vi "Elbow Call.vi"(3 "Button Values":bool[](array[boolean])) -> ()   [LabVIEW 2018]
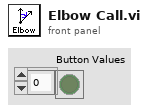
[diagram p1: front panel]
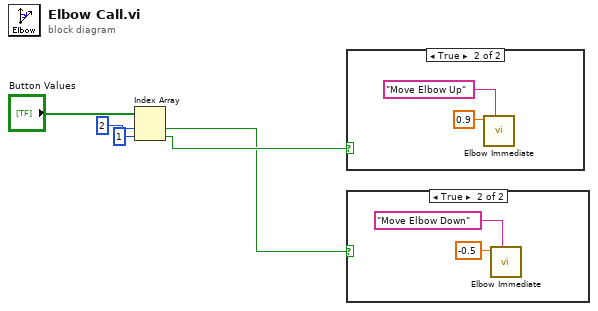
[diagram p0: block diagram]
diagram:
  n1 = Index Array(array="Button Values", index #1=2 ("index"), index #2=1 ("index")) -> (element #1=w1:bool, element #2=w2:bool)
  n2 = case shown="True" w2 {
    frame False {
    }
    frame True {
      n3 = call "Elbow Immediate.vi"("Description"="Move Elbow Up", "Setpoint"=0.9) -> ()  [unwired: 9 in, 1 out]
    }
  }
  n4 = case shown="True" w1 {
    frame False {
    }
    frame True {
      n5 = call "Elbow Immediate.vi"("Description"="Move Elbow Down", "Setpoint"=-0.5) -> ()  [unwired: 9 in, 1 out]
    }
  }
